vi "Connect List.vi"(8 "error in (no error)":errorcluster, 10 "Params":variant, 11 "PIPXI40 Matrix in":refnum<class "PIPX40 Matrix.lvclass">) -> (0 "error out":errorcluster, 3 "PIPXI40 Matrix out":refnum<class "PIPX40 Matrix.lvclass">)   [LabVIEW 2020, in "Pickering.lvlib" / "PIPX40 Matrix.lvclass"]
uses:
  PIPX40 Matrix.lvclass
  D:/WSGitHub/RTFWK/Realization/PIPX40 Base/PIPX40 Base.lvclass
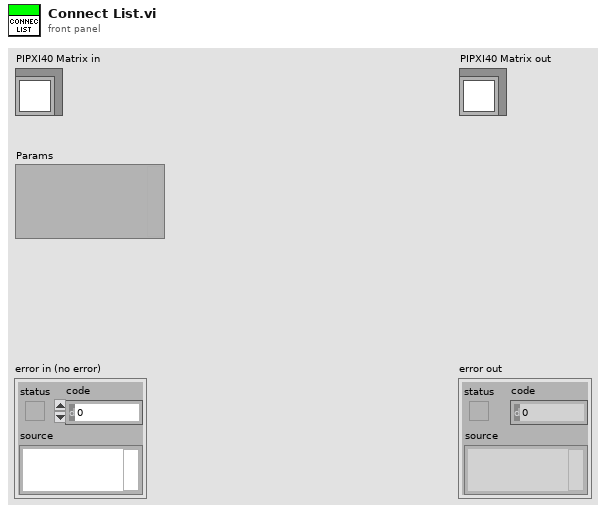
[diagram p1: front panel]
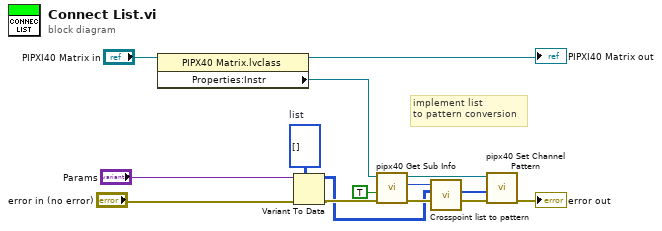
[diagram p0: block diagram]
diagram:
  w14 = i32[][] []  # list
  # "implement list\nto pattern conversion"
  n1 = property class="PIPX40 Matrix.lvclass"(reference="PIPXI40 Matrix in") -> (reference out=→"PIPXI40 Matrix out":refnum<class "PIPX40 Matrix.lvclass">, "Properties:Instr"=w6:refnum<visa-resource-name>)  [unwired: 1 in, 1 out]
  n2 = Variant To Data(error in="error in (no error)", type=w14, Variant="Params") -> (data=w2:i32[][], error out=w7:errorcluster)
  n3 = call <instrlib>:"pipx40 Get Sub Info.vi"("error in (no error)"=w7, "is output"=TRUE, "instrument handle"=w6) -> ("error out"=w8:errorcluster, "rows"=w1:u32, "instrument handle out"=w9:refnum<visa-resource-name>)  [unwired: 4 in, 2 out]
  n4 = call "Crosspoint list to pattern.vi"("List"=w2, "rows"=w1) -> ("Pattern"=w3:u32[])  [unwired: 9 in]
  n5 = call <instrlib>:"pipx40 Set Channel Pattern.vi"("error in (no error)"=w8, "pattern"=w3, "instrument handle"=w9) -> ("error out"=→"error out":errorcluster)  [unwired: 7 in, 1 out]
